vi "CALCULADORA AERODINAMICA.vi"() -> ()   [LabVIEW 2019]
panel:
  in  "Combo Box":string(combo)
  out "DENSIDAD":dbl
  out "PRESION":dbl
  in  "stop":bool
  out "TEMPERATURA":dbl
  in  "Altitud":dbl
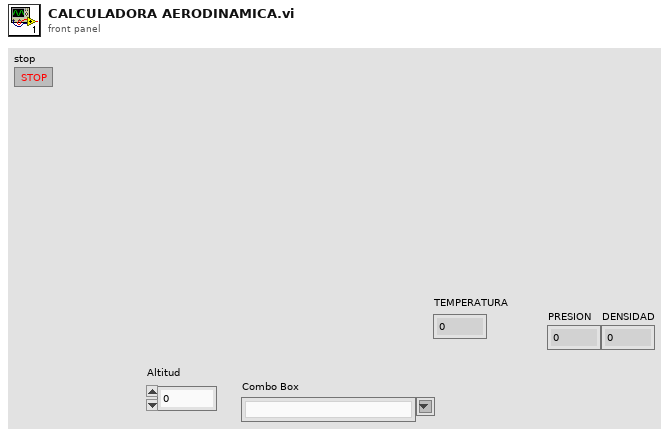
[diagram p1: front panel]
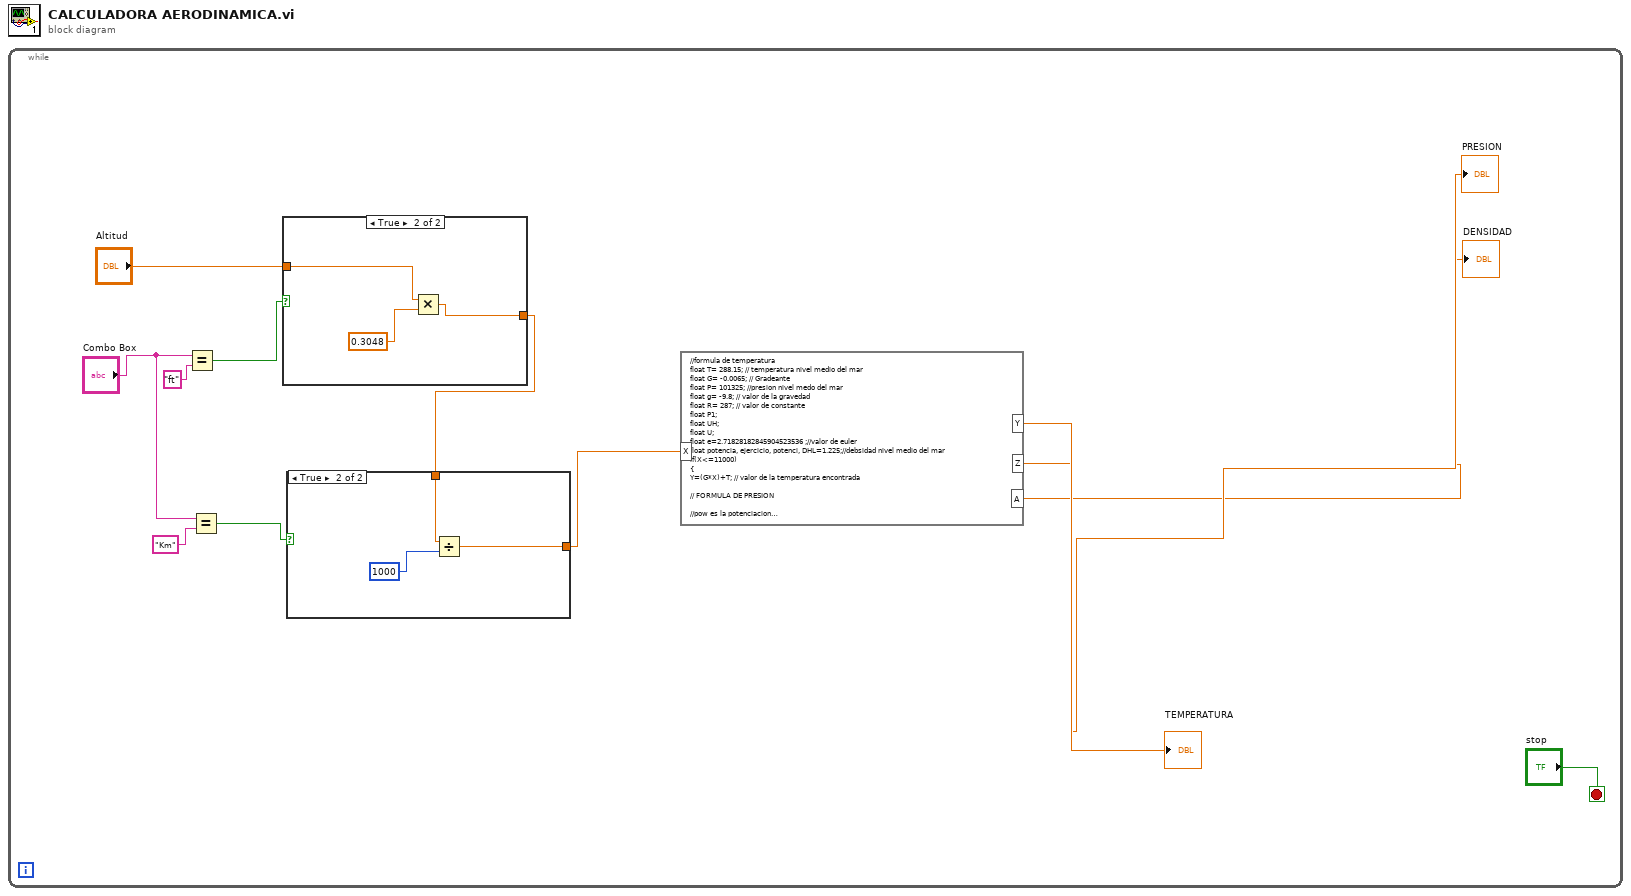
[diagram p0: block diagram]
diagram:
  n1 = while {
    stop <- "stop" stop-if-true
    n2 = Equal?(x="Combo Box", y="ft") -> (x = y?=w10:bool)
    n3 = Equal?(x="Combo Box", y="Km") -> (x = y?=w7:bool)
    n4 = case shown="True" w10 {
      tunnel: "Altitud" -> [w17 w20]
      tunnel: [w17 w18] -> w5
      frame False {
      }
      frame True {
        n5 = Multiply(x=w20, y=0.3048) -> (x*y=w18:dbl)
      }
    }
    n6 = case shown="True" w7 {
      tunnel: [w13 w15] -> w4
      tunnel: w5 -> [w13 w14]
      frame False {
      }
      frame True {
        n7 = Divide(x=w14, y=1000) -> (x/y=w15:dbl)
      }
    }
    n8 = formula code="//formula de temperatura\nfloat T= 288.15; // temperatura nivel medio del mar\nfloat G= -0.0065; // Gradeante\nfloat P= 101325; //presion nivel medo del mar\nfloat g= -9.8; // valor de la gravedad\nfloat R= 287; // valor de constante \nfloat P1;\nfloat UH;\nfloat U;\nfloat e=2.71828182845904523536 ;//valor de euler\nfloat potencia, ejercicio, potenci, DHL=1.225;//debsidad nivel medio del mar\nif(X<=11000)\n{\nY=(G*X)+T; // valor de la temperatura encontrada\n\n// FORMULA DE PRESION\n\n//pow es la potenciacion \nejercicio=Y/T;\npotencia=g/(R*G);\nZ=P*(pow(ejercicio,potencia));\n\n//ECUACION DE LA DENSIDAD\n\n\npotenci=g/(R*G)-1;\nA= DHL*(pow(ejercicio,potenci));\n} \n// formula para encontrar depues de los 11000 m\n\n\n\n\nif (X>11000) \n{\nY=T+(G*11000);//TEMPERATURA DE LA FRONTERA\nejercicio=Y/T;\npotencia=g/(R*G);\nP1= P*pow(ejercicio,potencia);//PRESION EN LA FRONTERA\n\nUH= (g/(R*Y))*(X-11000);\nZ=P1*pow(e,UH);\nA=Z/(R*Y);//ECUACION DE LA DENSIDAD\n}"("X"=w4) -> ("Y"=→"TEMPERATURA":dbl, "Z"=→"PRESION":dbl, "A"=→"DENSIDAD":dbl)
  }
